vi "18_1.vi"() -> ()   [LabVIEW 2018]
panel:
  out "Array":u64[](array[numeric])
  out "sum":u64
  in  "Input":string="(7 * (7 * 6 * 4 + 3)) * 3 + ((8 + 5 * 3 + 7 + 8) + 3 * (2 + 9 * 5 + 7 * 5 * 6) * 2 + 3 * 9) + (4 + 5 + 5 * 2 + 2) + ((5 + 6 + 9 + 6) + 3 + 4 * 6 * 5)\n7 * 5\n(9 * (9 + 7) * 7 + (4 + 5 * 5 + 2 + 3) + 3) * 7 * 5 + 8 + (4 + (7 + 9 + 6 * 9) * 2)\n((6 + 4) * 6 * (5 + 3) * 9 * (3 * 5 * 5 * 9 * 4 + 9) * 4) * 2 * 8 + 9\n7 * 7 + (9 + 2 * 9 + 9)\n9 + (7 * 7 * 5 * 9 * 7) * 2 + 3 * 3\n5 * (5 * (8 * 4) * 7 + 8 + 7) * (5 * (4 * 3 * 5 + 2 * 5) + (6 * 6 * 7 * 2 + 2) + 4) + (5 + 4 * 7 + 5 * 9 + 9) * 2\n((7 + 3 + 8) + (2 + 6 * 4 * 5)) + 8\n8 * (6 * 7 + 3 * (8 * 5 * 2 * 4)) * (3 + (5 + 5 + 6) * (4 * 3 + 7 * 5 + 7) + (3 * 5 * 9 * 3)) + 8\n6 + 4 + 8 + 4 * ((3 + 5 * 8) + 7 * 7 * 8 * 7 * 2)\n3 * (9 + 4) * (9 + 2 + 6 + 5) + 4 * (7 * 2) + 6\n4 * 6 + (8 + 3) + 7\n2 + (8 * (5 + 6 * 5) + 9 * 7 + (7 * 7)) + 5 + 5\n(8 + (5 * 7 * 3 + 6) + 8) * 8 + 6\n8 * 6 * 6\n8 * 6 + (9 + 4 * 5 * 3) * 9 * (4 * 2 + 6 + 7 + 4 * 8)\n(5 * 9 * 8 * 9 * 6) * 8\n7 * 5 + ((2 * 7 * 5 + 2 + 6 + 3) * 9) * 5 + ((2 * 2 * 4 + 3) * 5)\n(2 + 3 * 4 * (2 + 4 * 9 + 8) * 8) + 6 + 8 + 7 * 2\n3 + 7 + (3 * 4 * (8 * 6 + 8 * 8 * 2 + 9)) * 4\n9 * 9 + 9 + (3 * 7 * 9 * 4)\n(7 * 7 + (2 * 5 * 8) * 4) * 9 + (9 + 4 * 8 * (9 + 3 * 5 * 4 * 7 * 4)) + 3 * 3\n7 + 6 + 3 * 8 * 4 * (9 * 4 * (5 + 7 * 2 * 8 + 7 * 8))\n(7 + 2) * 5 * 8 + 6 * 2\n9 + 4 + (5 + (7 * 7 * 9 + 5) + 6 * 5 + 2 * (4 * 7 * 7 + 8 * 5 * 5)) * 2 + 2\n8 + 2 * 2 * (2 + (2 + 7 + 7 * 7 * 3) + 7)\n3 + 4 * (3 + 3 * 3 + 4) * 9 * 6 + 8\n((4 + 4 + 6) + (5 * 5 + 4 * 9 * 5) + 5) + 2 * 2\n9 * 5 * 6 * 2 + 6 + (2 * 9 + (2 * 3 + 4))\n(3 * 9) + 2 * (2 * 5 + 7 + 9 * 7 * 6) + 5 * 5 * 2\n7 + 3 + 5 * 6\n7 + 5 + (2 * 8 + (6 * 6) + 6) + (4 + 7)\n2 * (9 + 5 * 3 + 5 + 5 + 4) * (3 + 4 + 3 + 5 + 2 + 7) + 2 * 2\n(4 * 5 + 6 * 3 + (5 * 3)) * 5 + 5\n9 + 8 + 7 * (7 + 9 + 2 * 2 + 7) * 7\n3 * 3 * ((4 + 3 * 4 * 2 * 2 * 6) * (9 + 6) * 3) * 5\n9 + 6 + 7 + 6\n8 * (4 * 8 * 8 * 7 + 4 + 9)\n2 + (7 * 9 * 2) + 6 * 6 * 4 * 6\n((4 * 6 + 7 + 9 * 4) + 9) * 4 * ((6 * 3 + 3 + 9 * 7) * 8 * 4 * 5 * (2 * 6 * 8 * 5 + 5 * 3)) * 7\n(4 * 7) + 5\n6 + 9 * 6 + 9 + ((5 + 7 * 5 * 8) + 7 + 7 + 8 * (2 + 8 * 2 * 4 * 7 + 9) * 7)\n6 + 3 + (9 + 6 * (4 + 7 + 4 * 6 * 7)) + 6\n5 * 7 * (4 * 6 * (3 + 8 + 6 * 8)) + 8\n(5 * 6) * 8 + 2 * 3 + (7 + 4 + 3)\n3 + 4 * 9 * 2 + (7 + (5 * 9 * 7 + 7 * 4) * 4) + 3\n2 * 9 + ((3 + 5 + 2 + 9 * 9 + 6) + 4 + (6 * 4) + 2) + 3\n3 + 6 + (3 + 6 + 8 + 2 + 2)\n8 * ((8 * 6) + (7 + 2 * 2 * 2 + 4 * 3) * (9 + 8 + 4 * 8) + 8 * 4) + 2\n9 + 4 * (7 * (2 * 4 + 9 * 3 + 7) * 8 + (4 * 3 * 9 + 9 * 5 + 7) + 9 * (6 * 4 * 2)) + ((5 + 6 + 7 * 9 * 6 + 6) + (6 * 2 + 8 + 9 + 4 + 4) + (8 * 5 * 2 + 6 + 7) * 5 + 3) * 9 * 8\n9 + 2 + (5 + 3 * 2 * (7 + 4 * 5 * 5 + 3 * 7) * 8 * (5 * 6))\n7 * (3 + 3 + 7 * 7 * 9) + (2 + 5 * 6 * 4)\n9 + 8 + 9\n8 * (7 + (5 * 7) + (7 + 3) * 2 + 7) + 4 * 3\n2 * (2 * 6 + 5 * 7) * 2 + (3 + 3) * ((2 * 3 + 2) + (5 * 3 * 4 + 8 * 2))\n4 * (3 + 7 + 6 + 8 + 3 + 6) + 8 + (2 * 3 * (5 * 2 + 6 + 5 * 8))\n2 + 5 + 3 + 2 + 4 + (2 + (6 + 4) + 5)\n2 * (4 * 4) + (5 + 2 * (4 + 2 * 2 + 4) * 4 + (5 * 9 * 9) + 2)\n(6 + 9 + (3 + 5 * 3) + 4 * 2 * 2) + 7 + ((6 * 6 + 4 * 5 * 5 + 4) + 5) + ((8 + 4 + 9 * 8 * 9 + 2) + (7 + 2 + 9) + 4) + 5\n7 * 3 + (6 + (8 * 5) * 6 * 8) * 2 * 9 * 4\n9 + 9 + 9 + 2\n(7 * 9 * 2 + 8 * 7 * 4) + 9 + (9 * 6 * 9 + 7) * 3 * (9 * 5 * 5)\n4 * 7 * ((7 + 9 * 5 * 4 + 7 * 4) + (2 + 3 + 5 * 4 + 2) + (2 + 5 * 8 * 5 * 5 + 6)) * 6\n5 + 8 * (9 + (9 + 3 + 9 + 5 + 5))\n(3 * 7 * 2 * 3 + (8 + 8 + 3 * 9)) + 8 + 8 * 6 + 8 + 6\n9 + 4 + 8 * (7 * 8 + 8 + 4 * 8)\n2 * 9 + 2 * (5 + 3) * 2 * (5 * 5 * 8 + (3 + 4 + 4 + 5) + 4 * 4)\n5 * 7 + 2 * ((2 * 8 * 8 + 8 * 2 * 7) * 6 * 7 + 7 + 2) * 2 + 9\n4 * (6 * (6 * 3 * 3)) * (7 * 5 * 4 * 2 * (5 + 5 + 8 * 3)) + 7 + 7 * 8\n3 * 2 + 4\n9 + 6 * 2 * 4 + 2\n((5 * 5 + 3 + 7 * 2) * 2 * 5 + (9 + 9)) + 3 + 6 * (9 + 8) * 8 * 9\n4 * (8 + 2 + 3 * 9 * 6) * 6 * 3\n2 * (9 * 6 + (8 + 6 * 4) * (5 * 5) + 9 * 2)\n6 + (3 * (6 * 6 + 4 + 5) + 3 * 5 * 4 + (6 + 9 + 4 * 5 * 3)) + 6 * (3 + (6 + 5 + 5 + 6) * 8 + 8 * 4) * 4 + 6\n9 * 9 * 2 + (6 * 4 * 2 + 4 * 7 * 9) * 7 + ((5 + 6 + 7 + 7) * (7 * 3 + 9) + 9)\n(2 + (6 + 8 + 6 * 5 + 5) + 8 * 5) * 9 + 3\n2 * 9 + 2 + (9 * (4 + 6 + 4 + 2) * 9 * 5 + 7 + 2)\n8 + 6 + 4 + 6\n3 + ((6 * 4 + 2 + 4 + 3 + 8) * (4 * 3) * (9 + 4 * 6 + 2 * 7 * 6)) + 5 + 7\n3 * (8 * 4 + 9 + 4) * 7 * 2 + ((5 + 9 * 6 * 4 * 4) * 8 * 4 * (6 + 2))\n((8 * 7 + 6) * 3 + 2 + 5) + 8 * 5 * 8\n(3 * 2 * 6 * 3 * 2) * 6 * 2 * 9\n(4 * 8 * 3 + 5) + (8 + 9) + 7 * 7 + 3 * 3\n(2 + 7 * (7 * 8)) + 8 + (6 * (4 * 8) * 4 * 2 * 8) * 4 * ((7 + 8 + 4 + 3 + 6) * 4 + 9 + 4) + 3\n((7 + 2 + 3 * 3) * 5 * 5 + 4) + 9 * 2 + 7 + 9 + 2\n(6 + (2 + 7)) * 4 + 7 + 8 * 5\n(9 * 8) + (8 + (2 + 4 + 5 + 6 * 9) + 2 * (8 + 9))\n2 * (9 + 8) * 8 * ((7 * 6 + 7 * 3) + 2 + 5 * (7 * 2 + 7 + 8) + 3 * 3) + 8\n4 * 6 + 6 + 4 * 9\n(2 + 4 + 5 + 3 + 6) + 3 * 3 * 3 + (5 * 2 * 9 + 6 * 6 + 5)\n7 * 5 + (6 + 2 * 2 * 8 + 5) * 6 + 6\n(5 + 8 + 2) + 3\n3 + 3 * 5 * ((3 + 8 + 5 + 9) * 4 + 4 * 4 + 4) + 8 * 3\n2 + (5 + 5 + (6 * 5 * 2 * 8) * 4 + 8)\n8 + (5 * 7 * 2 * 2) * (7 + 9 * 5) * 2 + 9 + 4\n((9 * 9) + 6 + 4 + 9) * 5\n5 + 3 * ((4 + 8) + 9 * 2 * 6 + 7)\n6 + 7 + 5 * (2 + 9 * 4 * 5 * 7 + 5) + 9 * 4\n(7 * 2 + 4 + (8 * 8 + 2 * 5 * 3 * 6)) + (4 + 4 * 3 + 7) + 4 * 6\n2 * (5 * 9 * (5 + 3 * 5) * 5 + 6) + 4 + 5\n5 * (4 + 7 + 4)\n9 * 7 + 8 + 4 + (6 * (6 * 2 * 4 + 9)) + 5\n6 * 3\n(5 * 6 + 2 * (2 + 5 * 6 * 4 + 9 + 2)) + (4 + 3 * (9 * 9 + 4 * 8 * 8 * 9) * 4) * (8 + 7 + (4 + 8 * 2 + 4) * 9)\n8 * 5 + 9\n7 + 4 * 9 * 6 + 6\n9 + 6 * (8 * (7 * 6 + 2 + 4 + 6 + 9) * 2 + 2 + 2 + (7 + 7 + 9))\n6 * (7 * 6 * 6) * 9 * 6 + 7\n(5 * 7 + 9) * 7 + ((4 * 5 + 3) * 5 * (3 + 8 * 7) + 2 + 3 * (7 + 6 + 2)) + (3 * 5 * 5) + 2\n4 * 2 * 2 * 2 * (6 + 4 + 9 + 4 * 5)\n((9 * 7 + 7) + 8 * 7) * 4 + (7 + 9 * 9) * 6\n8 * (6 * (8 + 4) + (5 + 6) * 6) * 7 + 4 * 7 * 2\n(7 + 7 * (8 * 5 + 4)) * 5 * (3 * 6 * 2 * 3 * 9) * 3\n4 + (7 * 5 * 3 * 5 + 3 * 5) * 7\n(6 + 5 + 6 * 3 * (6 * 4 + 6)) + 2 * 5 * 9 + 3 * 5\n3 * (6 + 3 + 5 * 3) + 6 * 3 + (7 + 8) * 9\n(3 + 8 + (5 * 4 + 4 + 7) + 5 * 2) + 2 + 5 + 6 * 9 + (4 + 2 + 6)\n9 * 8 + (3 + (4 + 2 * 8 + 7 * 5 + 3) + (3 * 3) * 3 + (2 * 8))\n7 * 4 + (3 + 7 + 6 + 4 * (3 * 6) * 2) + ((5 + 5 * 5) + 6 + 2 * (2 * 3 * 3 + 3))\n9 * 5 * (6 + (2 * 3)) + (3 * 4 + 3 + 9 + 6) + (9 + 5 + 2 + (3 * 4 * 9 * 9 * 5) + 2 * 7) * 5\n(6 + 9 * 4 + 5 * 4 * (8 + 2 * 4 * 2 * 3)) + 4 * 9 + 6 * (4 * 5 * 9)\n9 * 7 + (2 + (6 + 3) + (4 * 3 + 9) + 9) + 8 + 9 * 3\n3 * (8 + 7 + 7 + 8) * (5 + 5 + 2 + 6 + 9 + 7)\n7 + (7 * 5 + 3 * 4 * 9 + 2) * (8 * 6 + (5 + 2) + 6) * 4 + (6 * 3) + 2\n(4 * 5 + 7 + 3 * (7 * 8) + 8) + 6 * 2 + 9 + 3\n7 * 4 * 8 * (7 + 5 + 2) + (8 * 8 * 2) + 3\n7 + 7 * (6 + (4 * 7 + 3 + 2 + 7) + 3)\n2 + (8 + (5 + 9 + 2 * 6 * 6 + 8) * 8 + 2 * (5 * 2 + 8) * 4) + 2 * 6\n(4 * 9 * (7 * 6 * 9 + 8 * 6) * 9) * 2 * 2\n3 + (8 + 2 + (2 + 3 * 2) * 6 + (5 * 8 * 8 * 8 + 2 + 3)) * 4 * (9 + 3) * 6\n8 + 3 * (3 + 5) + 3 + 5\n4 + ((9 * 5 * 2 + 7 + 5) + 6 + 3 + 6 * (7 * 6) + 6) * 2 * 3 * (3 * 9 + 9)\n((4 * 9) * 8 * 6) + 8 * 8 + 6 + ((6 + 4 + 7) * (2 + 2 * 4 * 9) + 3 + (5 * 9 + 9 * 9 + 5) + 2)\n(8 * 4) + (8 + 8)\n((4 + 5 + 2 * 4 * 7 + 3) * 6 * (4 * 6 + 8) * 9 * (9 + 7 + 5 + 3)) * 5\n8 * 2 + 8 + (7 * (8 + 2 + 6 * 7 + 9) + (5 + 9 + 3) + 6 * 6) * (8 + (4 * 2 + 4 + 7 * 5) + 2 * 6) * 5\n(2 * 5 + (8 * 7 + 9 + 2 + 2)) * 2 + (8 * (2 + 4) + 4 * 5 + 7) + 4\n4 + (2 + (4 * 3 * 9) * 5 * 4)\n((3 + 4) * 7 + 6 + (5 * 3 * 8 + 8 * 9) * 3 + 6) + 8 * 4 * ((7 + 4 * 3) * (6 + 9 + 9 * 4 * 7) + 9 + 5 + 2 + (5 + 8 * 4 * 6 + 4 * 8))\n4 * (9 * 5 * (5 * 7 * 7 + 4)) * 5 * (5 * 7 + (4 * 5) * 4 + 9)\n5 + (8 * 6 + 8) + 8\n7 + (8 + 6) * 4 + 2\n(3 * (9 + 6 * 8)) * 8\n3 + 6 + 4 + ((5 + 4 * 2) + 7)\n7 * 3 + 5 * (2 * 5 + 4) * 8\n5 * 5 + (6 * (8 + 5) * 7) * 7 + 4\n7 + 9 + (2 + (3 + 8 + 4) + 9 * 2 + 6) * (7 + (3 + 6 * 8 + 8 * 7) + 9 * 3 * 8 + (9 * 6 + 2 + 8 + 4 * 4))\n6 * (2 * 8 + 3 + 5 + 5) + (3 + (8 * 2 * 3) * (2 + 9 * 8 * 5 + 3) + 4 + 7) * 7 + (5 * 5 + 7)\n(2 * 2 * 6 * 4 * 9 + (9 * 5 + 7 * 4 + 6 * 2)) * 4 + (4 + (8 * 2 + 3 + 6))\n2 + (8 + 4 * 8 + 3) * 6 + 7 + 4\n(6 + 6 * (2 * 5 * 5 * 4 * 5 * 4) + 8 * 7 * 3) + 5 + (3 * 6 + 3 * 7) + 5 + 5 * 3\n2 * (8 + 2 + 6 * (9 * 9 * 9 + 4 * 2 * 7) * 3 * (4 + 6 * 3 + 8 + 4)) + 8\n(6 * 7 + 8 * 6 * 7 + (5 + 9 * 3 + 6 + 9 * 5)) + 2 * 6\n(7 + 2 * 4 + 3) + 4 * 5 + 3\n((7 * 7 + 2 + 7) + (3 + 3 + 5 + 9 * 3 + 2) * (2 * 4 * 7 + 6 * 3)) * (2 + (7 + 4 + 3 * 9 + 4 * 5) * 4 + 3 * (5 + 8 * 3)) + 5 + (2 + 8 * 2 * 8 * (6 * 7 + 4 + 5)) * (3 * (7 * 6 * 3 * 8)) + 7\n3 * 4 * ((8 + 8 + 9) * 6 + 6 + 7 + 6) + 8 + 3\n(6 + (7 * 4) + (9 + 6 + 3 * 9)) + 2 * (4 + 6 * 5 + (2 + 8) * 5 + 9) + 3 * (6 + 8 + 8 * (7 * 8 * 3 * 2 + 2 + 8))\n(9 + 8 * 4 + (5 * 8 + 7 * 2 * 8 * 9) * 8 + 9) * 3\n9 + ((5 * 3 + 6) + (8 + 6 * 6 + 7 + 2 + 8) * 8 + 5 + (9 + 8 + 2 * 9 + 2)) * 7\n((8 + 2 + 6 + 3) * 8 + 5 + 8 + 2) * 9\n(6 + (4 * 4 * 7 * 2 + 6) * 4 + 2 * 8 * (6 + 2 * 8)) * 2 * 8\n3 * (4 + 3 + 3 + (3 * 7 * 7)) + 6 + 7 + 4 + 8\n(6 * 8 + 7) * 8 * 9 + 8 + 4\n(7 * 7) * 2 + (8 * 7) + 4 * (5 * 2 * (3 + 4 + 7 * 8 * 3) * 9) + 6\n7 + (9 * (6 + 8 * 7 + 6 * 3) + 4) * 4 + 3\n6 + 3 * ((2 + 2 + 3 + 9 + 9 + 8) * 6 + 2) + 5\n3 * 6 * 6 + 2 + 2 + (2 * 2)\n6 + (4 + 9 * (5 + 9 * 4 * 6 + 6) + 4 * 6 * (2 * 7 * 7 * 4 + 8)) + 5\n((2 + 6) + 2 + 5) + 7 + 3 + 5 * 3 + 5\n(6 * (2 + 8 + 7) + 4 * (2 + 8) * 9) + 9 * 6\n(2 * (9 * 4 * 3 * 2) + (4 + 4 * 3 + 2)) + 4\n(6 + 4 * (5 + 9)) + 7 * 7 * 8 * 5 * 3\n(3 + (5 + 4 * 3 + 9)) * 2 * (9 + 6 * 6 * (7 + 8 + 2 * 5) * 8 * 6)\n8 + 6 * 6\n8 + (8 * 9) + 5\n8 + (7 * (6 + 8) * 7 * (5 * 7 * 8 * 7) + (8 + 4 + 6 * 9 + 8) + 4) + (6 * 4) * 3 * 7\n9 + 4 + 3 * 7 * 5\n(8 + 9) + 6 + 4 * 7\n5 * (4 * 6 + 4 + 2 * (5 * 2 * 2 * 8)) * 3\n3 * 3 + 2 + ((8 + 5 + 4 + 8 + 8) * 7 * 6 + 9 * 8)\n9 + (8 + (8 + 9) + 7 + 8)\n(8 + 2) + (2 + 5 + 7) + 6 * 6 * 6 * 6\n5 + 7 + (5 + 4 * (5 * 6 + 3 + 3) + (7 * 9 * 5 * 6 * 6 + 3) * 8) * 7\n6 + ((7 * 3) * 6 * 5 + 5 + (3 + 3 + 9)) + (6 * 2 + 6 + 9 + (2 + 4 * 3 * 4) + 7)\n8 * 5 + (9 * 2 * 7 * 2 * 6 + 8) * 2 + 2 + 6\n6 * 8\n(2 * 3 + 5 + (8 + 6 * 8 * 7 * 2)) * 3 + 2 + 6 + 2 * 5\n(7 + 6 * (2 + 2 * 4 * 9 + 7 * 5) * 4 + 2) + 4 * (9 + 6) + (9 + 5) + 7\n5 * (3 + 7 + 7 * 4)\n2 * ((2 * 7 * 8 * 4 * 3 + 7) + 6 + 3) * 5 * 7\n8 * 4 + 7 + (6 * 4 + 3 + 2) + 7 * 8\n7 * 9 + (2 * 9 * 2) * 6\n8 + (6 * (2 + 8) + 9) + (7 + 6 + 6 * (8 * 3 * 5 * 5 * 9) + 3 + 7) + 8\n2 + 5 * 4 + (4 * (3 + 7 * 5 + 8) * 8 + 2) + 3 * 7\n(8 * (9 * 7 + 9 + 9 + 4) * 3 + 2) * 8\n4 + (6 + (2 + 4 * 6) + 4)\n(8 * (4 + 6 + 2 * 6 + 7)) * 9 + 8 + 3 * 5\n((2 * 7 + 3 * 5) * (5 + 7 + 7 + 3 * 7 * 3) * 8) * 2 * ((2 * 9 * 4 * 6 + 4) + 6 + (8 * 5 * 4 * 5 * 6 * 8) + 7 * (9 * 6 + 7 * 3 + 4 + 7)) + 9\n6 + 8 + (3 * 3 + 2) + 5 + 4\n5 * 6 + 6 * 5 * ((3 + 5 * 8 + 4 * 8) * 9 * 9 + 6 * 4 + 6) + (4 * 7 * 5 + 9 + 7)\n2 * 7 * (4 * 7 + (4 + 7 + 4 + 3 * 2 + 7) + 7)\n((8 + 3 * 6 * 6 + 4) + (9 + 5 + 3 * 3) + 7 * (3 * 4 + 4 + 9 * 4 + 6) + (8 + 5 + 2 * 2 * 5)) * 8 * 6 * 7 + ((5 + 6 + 2 * 4 + 2) * (9 + 8 + 9) + 6 + (6 * 5 * 9 + 7) * 4 * 6) * 7\n4 * 5 * (9 * 3) + (9 + 6 + 5 * 8)\n3 * 8\n9 + 2 * (7 + (2 + 9) * 9) + 4 * 4 * 8\n(8 + 4 + 7 * 2 + 8 * (8 + 7 * 4 + 4)) + 4\n4 + 8 + ((7 * 9 + 9) + 3 + 2 + 3) * 8\n(6 + (4 + 3 + 8 + 6 * 8)) * (5 + 9 * (5 + 2 * 7 + 8) + (6 * 7 * 4 + 2 * 5) + 4 * 9) * 8 * 5\n8 + 3 + 4 * 9 * ((4 * 9 + 3 + 6) + 3 * 3 + 9) * 2\n6 + ((3 * 2) * (4 + 9 + 9 * 5 * 2) * (2 * 8 + 4 * 7 + 4 + 8)) * 5 + (9 * 4 * 6 + 6 * 4 + 8)\n2 + (5 + 4 * 8) + (9 * 9)\n8 * 3 + 7 * 3 + ((2 * 2 + 6 * 3) * 3 * 7 * 8 + 5) + 9\n4 * 7 + ((6 + 7 * 3 * 4 + 8) * 2 + 6 + (4 * 6 + 9 + 6 * 8 * 3) + 3 * 3) + 3\n5 * (9 * 9 + (7 + 6 + 2 + 9 + 9 + 9)) * 8\n5 + 4 * 2 + 7 * (5 * 5 + 2 + 3)\n2 * 2 + 6 + ((2 + 2 + 5) * 6 * (2 + 7 + 3 * 9) * 5 + 9 * 8)\n((2 * 4 + 7) + 9 * 8) + 5 * 6 * 2 + 9\n6 + ((7 * 9 * 9 + 2) * 2)\n6 * (7 + (4 + 7 * 2) * 5 + 2 + 7) + 6 * 7 + 5\n8 * (6 * 8 + (7 + 2 + 7) + 3) + 7 + 6\n(7 * 2 * 3 * 7) + 4 * 3 + 6 * 9 + 7\n8 * 7 * (8 * 9 * 3)\n9 + (9 * 4 * (9 + 3 * 5 + 9 + 9) * 8 + 5 + 9)\n6 * (9 * 2 * 9 + 6 + 9 + 8) + (6 * 9 * 5) + 2 * 4\n2 * 5 * (7 + 8 + 3 + 8 + 6 * 4) * 4 + 5\n2 * 2 * (4 + 3) + 2 + 4 * 4\n(6 * (9 * 6 + 2 * 2) * 4 * 3 * 4 * 7) + 2\n(2 * 5) * 3 + 3 * 3 * 7 * 8\n3 + 6 + ((6 * 6) * (9 + 8 * 2) * 7 + 5 + 9 * 2)\n9 + 7 + (2 * 8)\n(8 * 7) + (8 + 6 * 7 + (3 * 9 + 6) * 6 + 8) + (4 * 2 * 9)\n2 + 2 + 2 + 9 * ((4 + 5 * 7 * 5 * 4 * 7) * (9 + 9) + 4 * 4 + 9) * 8\n4 + 2 + ((6 + 8 * 4 + 7) * 7 + 3 * 9 + (9 + 5))\n7 + 8 * (3 * (3 + 9 + 6 * 5) + 6 * 8) * 7 + 4\n8 + 7 * (2 * (5 * 7)) + (4 * 3 + 7)\n(2 + 8 * 7) + ((8 * 9 * 3 + 3 + 5 * 7) * 2 * (9 + 6 * 3 * 5) * 4 * (4 + 6 * 6 + 4 * 9) * 3) * 6 + 4 * 4 + 2\n3 * (9 + 4 + (9 + 5 + 8 + 6 * 3 * 4) * 8 + (9 * 3 + 8 + 4 + 7)) * 8\n(4 + 4 * (4 * 7)) * 2 + 7 * 3\n((4 * 9) * (9 + 6 + 9 * 8 + 7)) + 6 + 7 + 7\n6 + ((9 * 5 + 9 + 6 * 6 + 4) * 7 + (9 + 5 + 5) * 9 + 3) * (5 * 9) + 8 + 9\n(3 + 8 * (7 * 3 * 4)) * (6 * (6 + 4) + (9 + 8) * (2 * 5 + 4) + (8 + 5 * 6 + 5 * 2 + 2)) * 6 + 9 + (7 + 6 * 5) + (5 + 4 + (6 + 8 * 2) * 2)\n4 * ((6 * 8 + 7 * 6 + 4) + 4)\n((5 * 6) + 4) + (9 + 4 + 9) + 2\n5 * 9 * 7 * 6 + (9 * 7)\n5 + (2 + 7) * 5 + 9 + 7\n6 * 2 * 8 + 4\n(3 + 2 * 4 + 8) + ((7 * 5 + 7 * 2 * 8) + 7 + 2) * 6 * 2 + 5\n(2 * 5) * (3 * 9 * 4 * 8 + 5 * 3) * ((9 + 5 * 6 * 3) + 3 * 7 + 4) * 5\n((3 + 6 * 3) * (4 + 9 * 5 * 6 + 4 * 7)) + ((8 * 7 * 2 + 7) + 5 * 6) * 6 + 7\n(8 + 4 * 8 * 8) * 9 * 9 + 7 + 4\n(7 * 9 + 5) * 5 + (9 + 4 + 4 + (7 * 9 * 2 * 8 * 2 + 9)) * ((7 * 5 * 7 * 3 * 7) * 5 * 2) + 8\n5 + (6 * (8 + 9) * 7 + 9) + 3 + 3\n8 + 8 * (6 * 5 * (3 + 5 + 9 * 2 * 9 * 7))\n5 * (4 + 7) * 5 + 7 + 8 + 6\n3 * ((5 + 6 + 2 + 7) * 4 * 6) * 5 * 5\n(6 + 3 * (9 * 9 * 7 * 8 * 9 + 9) + 5) * 8 * 6 + 7 + 2\n8 * (4 + 3 * 5 + (5 + 2 * 3 + 8) * 2 + (8 + 7 * 7 + 4 * 7 + 7)) + 8 * 6 + 4 * 5\n4 + 7 * 8 * (2 + 6 + 5) * (4 + 8 + 4)\n9 + 8 * ((2 * 3 * 6 + 4 * 2) + (6 * 5 * 9 + 7) * 5 * 2 * 9 * 7) + (9 + 4 * (2 * 8 * 7) * 3 + (9 + 8)) + 3 + 6\n7 * 3 * 8 + ((6 + 7) * 9) * 2\n5 + 3\n4 + 9 * 7 * ((7 * 8 + 7 * 2 + 5 * 7) + 5 * 4) + (5 * 5 + (7 * 6) * 6)\n((2 + 4) * 5) * 3 + 5\n5 + (2 + 8 * 9 * 6 * 2 * (2 + 8 + 3 + 5)) * 9 * 8 + 3 * (9 + (4 + 2 + 4 + 7 * 4) * 9 * 9 + 7)\n2 + 6 * 9 + 3 + (7 + 8 + 2) * 4\n5 * 4 * (2 * 4 + 3 + 3 * (9 + 6 + 6) + (3 * 8 * 4)) * 4 * 3 + (9 * 7)\n7 * (5 * 5 + 4 + 8 + (3 * 4 + 6 + 9)) * 2 * 9 * (6 + 7)\n2 + (5 + 3 * 5 * 8) + 3 * 8 + (9 + 9 * 8 * 2 * 2)\n((7 + 9 * 9) * 7 * 2) + 6 * 6 * 9\n(6 * (9 + 9 + 4 + 5 + 6 + 2) + 6 + 8 + (7 * 3 * 8)) + 2 + 6 + 2\n(3 + (6 * 2 + 2 + 6 * 7 + 8) * 9 * 2) * ((2 + 9) + 8 * 9 + 2) + 3 * (3 + 4 * 7 * (3 + 2 * 8 * 6 + 7) * (5 + 3)) * 5\n(9 * (9 * 9 + 7 * 4) + (7 * 4 * 7 * 5) * (9 * 2 + 8 + 5 * 6)) * (6 * (7 + 9 + 6 * 7 + 9) + 4 * 4 * 2 + 6) * 9\n4 + (3 + (4 + 5)) + 7 * (6 + 4 * (5 + 3 + 9 + 5 + 2) * 4 + 4) + 8 + 8\n((5 + 8) + 5) * 9 + 6 + 8 * 7\n8 * (5 + (3 * 3 + 6 * 3)) * 5 + 2 + 8 * 8\n6 * 2 * 9 * (8 * 7 * (2 * 4 + 6 + 7 + 4 * 5)) + 9 + 7\n(5 * 3 * (8 * 2 * 8 + 2 + 8) * (8 + 8 + 9 * 7 * 6 * 3) + (4 * 2 * 7) * 4) + (4 * 3 + 9 * 5) + 5 + (5 + 9)\n(6 + 3) * 5 + (6 + 7 + 5 + 7)\n(9 * (6 + 6 * 8 + 4) * (3 * 6 + 6 + 7 + 7 + 5) + (5 * 7 + 4) * 9) * (7 + 3 + 7 * 2 + (5 + 7 * 6 + 8) * 4) * 7\n6 + 8 * (5 * 5 + (3 * 2 * 2 * 7 + 4 * 9) * 7 + 4) + 8 + 4\n9 + (5 * 7) * (5 * 6 * 8 * (5 * 2) + 9) * (6 + 3 + 6 + 9 + 2) * 6\n8 * (8 + 8 + 9 + 9 * 6 * 3) + 8 * (3 * 3) + 3 * 3\n7 * 7 * (5 + 5 * 9) + (6 * 6 * 3 * 4 * 8 + 8) + 3\n(3 * 2) + 5 * (6 * (9 + 2 + 3 + 2 * 9 + 5) + 6) + 2 + 7 * 9\n9 * 2 + 3 + (3 * 7) + 4\n7 * 5 * 7 * (4 + 3 * 7 + 3 + (4 * 5 + 5) + (5 * 8)) * (8 * 3 * (8 + 9))\n((3 * 8 * 8 + 6 + 5 * 5) + 3 + (3 * 8 * 7)) * 2 * (9 + (9 * 8) * 5) * 5 * 4 + 7\n4 * 9 * (4 + (3 * 7) + (6 * 4 * 9)) + 2 + 8\n5 * ((7 + 2 + 6 + 6) * 2 + 4 * 8)\n5 + 9 * ((7 + 2) * 5 * 4 * (5 + 7) + (8 + 4 * 8 * 7 * 9))\n((4 + 3) + 6 * 3) * (4 * (4 * 6) * 3 * 2 + 8 * 4) + 8\n5 + (6 + 3 + 6 * 8 * 7 * 2) + 3 * 9 + (8 + 2 + 6 * (4 + 6 * 6 * 8 * 3 * 3)) + 7\n7 + (8 + 8 * (8 + 3 * 3 * 5 + 2)) + 4 + (2 + 3 * 7 * 7 + 6 + 2) * 9\n7 * 3 * 2 + 6 + 7 * 4\n(3 + 4 * 7 + (8 * 3 * 5 * 8 + 5 * 3) * (7 + 4 * 8 + 9)) + 8 + (4 * 3 * 4) * (6 + 4 + 8) + 5 + (9 + 6 + 2 + 4)\n((3 + 9 + 5) * 7 * 2 * (3 + 7)) + 5 + 3\n(4 * 9 + 3 + 9) * 8 * 8 + ((7 * 2 + 6 * 2 * 2) + 8 * 3 * 2 + 2 + 6) * 3 + 7\n(5 * 6 * (8 + 8) + 2) + 6 + 2 * (5 + 4) + 2\n(3 * 8 + 2 + 5 + 6 + 6) + (8 + 7 + 9 * 4 * 4 + (4 * 4 + 4 * 7 + 7)) * 4\n(7 * 7 * 4) * 7 * 3 + 6\n(9 * 3 + 7) * 7 + 4 + 2 * 7 * 3\n6 * 9 + (6 * 6 + 6 * (3 * 9 + 7))\n5 + 6 * 7 + 8 + (3 * 3 + 5 + 3 + 6) + 8\n(6 + 4 + 6 * 9) + (3 * (6 * 3 * 2 + 2 + 9)) + (2 + 9 + 8 * 3 * 8 + 9) + 4 + (4 + 4 + 7)\n4 + 3 * ((6 * 3 * 2) + 3 * 3 + (6 * 4 + 5 * 5 * 7) * 6 + 3)\n2 + (7 * 5 * 6 + 8 + 4 * 8) * 3 * 6 * 3\n9 * (8 * (6 * 7 + 7) * 3 + 9) + 7 * 5 + 6\n((3 * 5) + 2 * 4 * 2) * 7 + (4 + (4 * 2 * 6) + 2) + (3 + 5 * 8 + 6) + (5 + 2 * 6) * 2\n8 + 9 * (4 + 6 + 9 + 2 + 4 + 6) * (9 + 4 * 5) * 2\n(6 + 9 + 4 + 7 * 7 + (6 + 5 + 4 * 6 + 4 * 5)) * 3 + 7 + (2 + 9 + 7 + 8 + 4 * 5)\n(6 * 7 * (7 * 7 + 3 * 9 + 4 * 2) + 8 * 7) * 3 * 2\n(7 * (5 * 2 + 2 + 8 * 4 + 6)) + 7 + 7 * 8 * 7 + 2\n(8 * 6 * (4 + 6 * 8 * 8)) * 8 + 4\n(4 + 7) * (7 * 4 + 4 + 5 + (9 * 9 * 4 * 5) + 8) + 4 + (8 * 9 + 2 + 4 * (2 * 2 + 8) * (5 * 7 * 4 * 6 + 2)) + 6\n4 * (8 * (2 * 5) + 4 * (7 * 2 + 7 + 8) * 7) * 4 * 9 * 7 + ((5 * 4 * 5 + 7 + 9) + 7 * 7 + (6 * 3 + 8 + 7 * 4) + (6 + 4 * 3))\n((3 + 4 + 7 * 8 * 5) * 9 * 6) + 6 + 3\n((7 + 3 * 8) * (3 * 7 + 4 * 3) + 5 + 2 * 9) * 8 + 4 + 2\n((3 + 8 * 8 + 9) * 5 * (5 * 6 + 5 + 7)) + 2 * (6 * 5 + 4 * 6 * 4 * 8) * 9 * 7\n4 + 9 * 8 * ((8 * 6) + 7 * 2 + 2 * 6)\n(2 * 3 * 3) + 4 * 8 * (3 * 5)\n(8 * (5 + 9) + (5 * 6 * 7 * 2) + 4 + 4 + (6 * 9 + 8 + 7 + 2)) * 7 * 2 * 6 + 2 * 2\n(8 * 9 * 7 + 3 * 6) + 5 + 4 * ((9 + 8) + (3 + 7 + 6 * 2) + (7 * 5 * 9 + 5) * 8 * 3) + (6 + 9 * (6 * 8) + 2 + 4 * 4)\n6 + 8 * 9 + (4 * (9 + 2 + 3 + 5 + 3 + 8) + (3 + 7 * 4) + 4 * 7 * (6 + 2))\n2 + 4 * 7 * 5 + (8 * 3) + 6\n9 + 9 + 4 + (4 * 3 + 3 * 2 + (7 + 2 + 9 + 8) + 4)\n3 * 7 * 7 * 9 + 7\n(3 * 2 * 3 * 5 + 6) + 4 * 5 + 8 + 5\n7 * 6 + 7 * 8 + 8 * 3\n(6 + 2 + (6 * 8 * 5) * 6 + 3 * (8 * 5 * 9 * 2 * 7 + 4)) * 3\n(8 + (4 + 2 * 3 + 7 * 5) * 9) * 3 + 9 + 4 + 6\n(9 + 6 + (6 + 3 * 2 + 8 * 5 + 7) + (8 + 8 * 3 + 9 * 4 * 8) + 6 * 2) * (7 + 9 + 5 + 8) * 7 + 4 * ((6 * 5 * 7 + 7 * 9 * 3) + (2 * 4 + 4 * 2))\n(5 * (3 + 5 + 5 * 6) * 7) + 8 + 3 * 4 + 7\n3 * 7 * (9 * 5 + 9 + 7) + 9 * (3 * 4 * 4 * (8 * 4 + 2 + 5)) + (9 * (5 * 3 * 4 * 9) + 5 * 8 + 9 * 5)\n6 + 7 + ((2 * 4 * 5 + 7) * 2 * (8 + 8 * 4 * 3) * 3) * 5 * 6 * 4\n7 * (9 * 6 * 4) + 7 + (8 * 2 * 7 * 4 + 8)\n4 + 7 * (8 * 4 * 2 * (2 + 5 + 9 + 5 * 2 + 5) * (5 * 6 + 2 * 5 + 9) + 3) * 9 * (3 * 6 + 3 * (4 * 4 * 6 + 6 * 2 * 9)) + 8\n2 + 6 * (8 + 9 + 6 + 2 * (9 + 4 * 7 * 5 + 5)) * (7 * 7 * 2 * 9)\n4 * 3 + (8 * (6 * 8 + 8 + 6) + 3) + 5\n(5 + 6) + (2 + 6 + 4 + 8)\n(9 * 5 * 3 + 6 * 6) + (5 * 4)\n3 * 2 + (7 + 7 * 2 + (6 + 6 + 2 * 8 * 4) * 3) * 8\n(4 * 6 + 6) + 4 * 9\n6 + (9 * 3 * 3 * 3) + 8\n(5 + (9 + 6 + 3 + 7 * 3 + 5)) + 5 + (4 * 3 + 4) * 9 * 3\n(6 + 8 * (8 + 3 * 2 + 4 + 5 + 9)) * 7\n6 + 3 * 3 * 5 + ((7 + 4 * 8) + 2 * 7 + 4 * (5 + 8) * 8) + ((5 * 4 * 2) * 4 * 5 + (3 + 4 + 4 * 7 + 7))\n2 * 3 * 3 * 4 * 7 + 2\n6 * (7 + 9 * 9 + (9 * 6) + 5) + 4\n8 * (2 * 7 + 5 * 5 + 8) + 5\n(4 * 5) + (3 + 3 * (5 * 9 + 8 * 2) + 6 * 4 + 4) * 5 + 6\n4 * 9 + (3 + 3 * 2 + (2 + 4 * 4 * 7 * 7 + 5) * 9) * 5 * 3\n(5 * 3 * 6 + 8 + 2 + 4) * 6 * 8 * ((6 * 2 + 2 * 4 + 6 * 2) * 6)\n4 * (5 * 4 * 6 + (7 + 3 * 9 + 3)) + (3 * 4 + 4 + (5 + 7 * 6 * 2 + 7) + 3)\n3 * (5 + 2 * 6 + 8 + 5) + ((8 + 3 * 6 + 8 * 3) * (7 * 7)) + 8 * 4 * 5\n4 + (8 + 6 * (4 + 3)) * 4 + 4\n4 * 3 * (3 + (8 * 9) * (9 * 7 * 4 * 9 * 4 * 8) * (5 + 2 + 2 + 2))\n8 + (2 + 2 * 5 * 3 * (4 * 3 + 7 + 6 + 3)) + 7 * 2 * 5 * 5\n4 * (7 * 9 * (2 * 2 * 5) + 2 + 8 * (6 + 2)) * 4 * 7 * 8\n(2 * 3 * 3 * 2 + (9 * 8 + 5 + 4)) + 7 * 2 * 6\n((6 * 7 + 3 + 3 * 4) * (5 + 9 + 5) + 7 * 6) + 9\n6 * 9 + 8 + 3 + 6 * (6 * 9 + 9 + 3 * 2 * 2)\n(3 * 5 + 2 + 9) * (6 + 9 + (6 * 8 + 2 + 8 * 3 + 8) + (2 + 6 + 6 + 6 * 3)) * ((7 * 5 * 9) * 3 + 9 + 3 + 8 * 2) * 8 * 6 + 8\n3 * (4 + 4 + 6 * (5 + 7) * 8) * (3 * (6 * 7 + 3 + 7 + 7) + 7)\n6 * 8 + 8 * (6 + 9 + 5) * 7 + 7\n3 * (8 + 5 + 8 * 7 * 7 * 8) + 7 + 9 * 4 + 9\n(4 + 5 + 7 + 6) * (9 * (6 * 3 + 9 + 3 + 3) + 6 * 8 + (2 * 8 * 4 + 7 + 5 * 4))\n7 * 2 + 3 * (5 + 9) + 7 * 3\n7 * 8 + 5 + 7 * 4 * ((7 * 4 + 8 * 8) * (6 + 5 * 8 + 7 + 5 * 3))\n(7 * 4 + 3) + (7 + 9 * 7 * 9 * (3 + 2 * 2 * 8 * 2 * 6)) + 5 * 3 + 3 + 3\n5 + 6 * (3 + 6) * (6 + (7 + 2) * 3 + (8 * 6 + 3 + 8 + 5 * 9)) * 7\n(9 + 6 + 8) + 3 + 5 + 2 + (3 * 9 + (8 + 3) + 7 * 3)\n6 + (9 + 7 * 2 * (8 * 9 * 2 + 7 + 6 * 7) * 6)\n2 + 4 * ((7 * 2 + 4) * 8) + 9 * 3 * 3\n3 + ((5 + 4) * 4 * 7 * (3 + 5 * 4 + 3) + 3)\n(7 + 4 * 3 * 6 * 7 * 5) * 2 * 7 + 4\n(7 * (7 * 9) + 8 + 2 * (6 + 9 + 9 * 2 * 5) + 7) * 7 * 7 + 9\n(2 * 5 + 9 * 5) * 3\n3 * 9 + 5 + 7 * 9 + 6\n9 * 3 * ((3 * 6 + 4 + 8) + 9 + 2) * 3\n8 * 3 + 6 * 8 * 2 + 4"
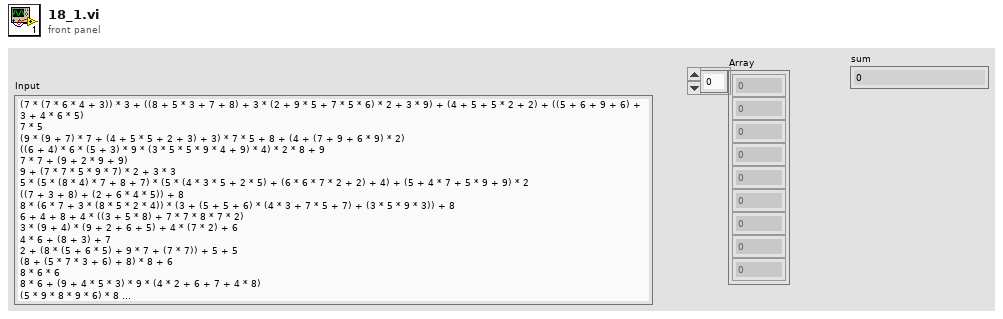
[diagram p1: front panel]
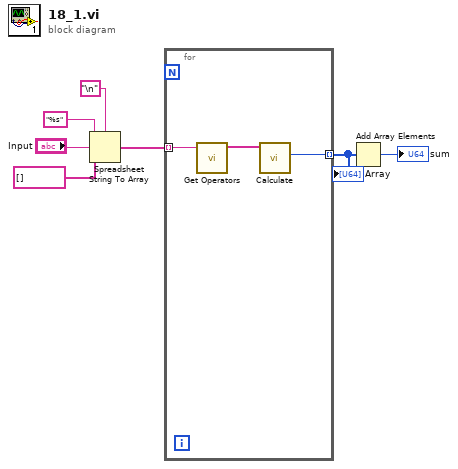
[diagram p0: block diagram]
diagram:
  n1 = Spreadsheet String To Array(delimiter (Tab)="\n", format string="%s", spreadsheet string="Input", array type (2D Dbl)=string[] []) -> (array=w3:string[])
  n2 = for {
    tunnel: w3 -> [w10] mode=indexing
    tunnel: [w8] -> w2 mode=indexing
    n3 = call "Get Operators.vi"("Expression"=w10) -> ("Operators"=w9:string[])  [unwired: 10 in]
    n4 = call "Calculate.vi"("Operators"=w9) -> ("Value Out"=w8:u64)  [unwired: 9 in, 1 out]
  }
  "Array" <- w2
  n5 = Add Array Elements(numeric array=w2) -> (sum=→"sum":u64)
